vi "publishHeartBeat.vi"(8 "error in (no error)":errorcluster, 11 "MonoCommunicator in":refnum<class "MonoCommunicator.lvclass">) -> (0 "error out":errorcluster, 3 "MonoCommunicator out":refnum<class "MonoCommunicator.lvclass">)   [LabVIEW 2016, in "MonoCommunicator.lvclass"]
uses:
  MonoCommunicator.lvclass
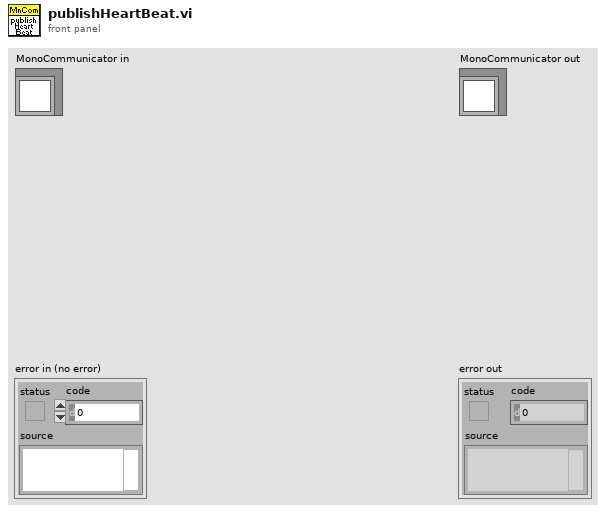
[diagram p1: front panel]
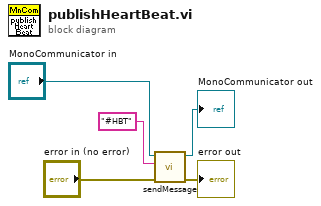
[diagram p0: block diagram]
diagram:
  n1 = call-dynamic "sendMessage.vi"("error in (no error)"="error in (no error)", "message"="#HBT", "MonoCommunicator in"="MonoCommunicator in") -> ("error out"=→"error out":errorcluster, "MonoCommunicator out"=→"MonoCommunicator out":refnum<class "MonoCommunicator.lvclass">)  [unwired: 7 in]
